vi "ProfiledPIDController_Calculate_Meas_StateGoal.vi"(9 "GoalState":T1 {"Velocity" format="%16_6e"; "Position" format="%16_6e"}, 10 "PV-Measurement":dbl, 11 "in PROFILED_PID_CONTROLLER":T2={"Controller"={"Kp"=0.0, "Ki"=0.0, "Kd"=0.0, "Period"=0.0, "Max_Integral"=1.0, "Min_Integral"=-1.0, "Max_Input"=0.0, "Min_Input"=0.0, "Continuous"=FALSE, "PositionError"=0.0, "VelocityError"=0.0, "PrevError"=0.0, "TotalError"=0.0, "PositionTolerance"=0.05, "VelocityTolerance"=9.99e+35, "SetPoint"=0.0, "Kf"=0.0, "Prev_Deriv"=0.0, "Prev_Deriv 2"=0.0, "DerivativeFilter"=FALSE, "Min_Output"=-9.99e+35, "Max_Output"=9.9e+35, "Prev_F_P"=0.0, "Prev_F_P_2"=0.0, "AntiWindupActive"=FALSE}, "Goal"={"Position"=0.0, "Velocity"=0.0}, "Setpoint"={"Position"=0.0, "Velocity"=0.0}, "Constraint"={"MaxVelocity"=0.0, "MaxAcceleration"=0.0}} {"Constraint"."MaxAcceleration" format="%16_6e"; "Constraint"."MaxVelocity" format="%16_6e"; "Setpoint"."Velocity" format="%16_6e"; "Setpoint"."Position" format="%16_6e"; "Goal"."Velocity" format="%16_6e"; "Goal"."Position" format="%16_6e"; "Controller"."Prev_F_P_2" format="%16_6e"; "Controller"."Prev_F_P" format="%16_6e"; "Controller"."Max_Output" format="%16_6e"; "Controller"."Min_Output" format="%16_6e"; "Controller"."Prev_Deriv 2" format="%16_6e"; "Controller"."Prev_Deriv" format="%16_6e"; "Controller"."Kf" format="%16_6e"; "Controller"."SetPoint" format="%16_6e"; "Controller"."VelocityTolerance" format="%16_6e"; "Controller"."PositionTolerance" format="%16_6e"; "Controller"."TotalError" format="%16_6e"; "Controller"."PrevError" format="%16_6e"; "Controller"."VelocityError" format="%16_6e"; "Controller"."PositionError" format="%16_6e"; "Controller"."Min_Input" format="%16_6e"; "Controller"."Max_Input" format="%16_6e"; "Controller"."Min_Integral" format="%16_6e"; "Controller"."Max_Integral" format="%16_6e"; "Controller"."Period" format="%16_6e"; "Controller"."Kd" format="%16_6e"; "Controller"."Ki" format="%16_6e"; "Controller"."Kp" format="%16_6e"}) -> (1 "CO-ControlOutput":dbl, 3 "out PROFILED_PID_CONTROLLER":T2={"Controller"={"Kp"=0.0, "Ki"=0.0, "Kd"=0.0, "Period"=0.0, "Max_Integral"=1.0, "Min_Integral"=-1.0, "Max_Input"=0.0, "Min_Input"=0.0, "Continuous"=FALSE, "PositionError"=0.0, "VelocityError"=0.0, "PrevError"=0.0, "TotalError"=0.0, "PositionTolerance"=0.05, "VelocityTolerance"=9.99e+35, "SetPoint"=0.0, "Kf"=0.0, "Prev_Deriv"=0.0, "Prev_Deriv 2"=0.0, "DerivativeFilter"=FALSE, "Min_Output"=-9.99e+35, "Max_Output"=9.9e+35, "Prev_F_P"=0.0, "Prev_F_P_2"=0.0, "AntiWindupActive"=FALSE}, "Goal"={"Position"=0.0, "Velocity"=0.0}, "Setpoint"={"Position"=0.0, "Velocity"=0.0}, "Constraint"={"MaxVelocity"=0.0, "MaxAcceleration"=0.0}} {"Constraint"."MaxAcceleration" format="%16_6e"; "Constraint"."MaxVelocity" format="%16_6e"; "Setpoint"."Velocity" format="%16_6e"; "Setpoint"."Position" format="%16_6e"; "Goal"."Velocity" format="%16_6e"; "Goal"."Position" format="%16_6e"; "Controller"."Prev_F_P_2" format="%16_6e"; "Controller"."Prev_F_P" format="%16_6e"; "Controller"."Max_Output" format="%16_6e"; "Controller"."Min_Output" format="%16_6e"; "Controller"."Prev_Deriv 2" format="%16_6e"; "Controller"."Prev_Deriv" format="%16_6e"; "Controller"."Kf" format="%16_6e"; "Controller"."SetPoint" format="%16_6e"; "Controller"."VelocityTolerance" format="%16_6e"; "Controller"."PositionTolerance" format="%16_6e"; "Controller"."TotalError" format="%16_6e"; "Controller"."PrevError" format="%16_6e"; "Controller"."VelocityError" format="%16_6e"; "Controller"."PositionError" format="%16_6e"; "Controller"."Min_Input" format="%16_6e"; "Controller"."Max_Input" format="%16_6e"; "Controller"."Min_Integral" format="%16_6e"; "Controller"."Max_Integral" format="%16_6e"; "Controller"."Period" format="%16_6e"; "Controller"."Kd" format="%16_6e"; "Controller"."Ki" format="%16_6e"; "Controller"."Kp" format="%16_6e"})   [LabVIEW 2019, in "Trajectory_Library.lvlib"]
doc: "Returns the next output of the PID controller.\n\nInputs:\n - Profiled_PID_Controller -- Profiled_PID_Controller data cluster\n - measurement -- The current measurement of the process variable.\n - goal -- The new goal of the controller.\n\nOutputs:\n - Profiled_PID_Controller -- Updated Profiled_PID_Controller data cluster\n - CO-ControlOutput -- Calculated PID output"
uses:
  Trajectory_Library.lvlib
  PID_CONTROLLER.ctl
  TRAPEZOID_PROFILE_STATE.ctl
  TRAPEZOID_PROFILE_CONSTRAINT.ctl
  PROFILED_PID_CONTROLLER.ctl
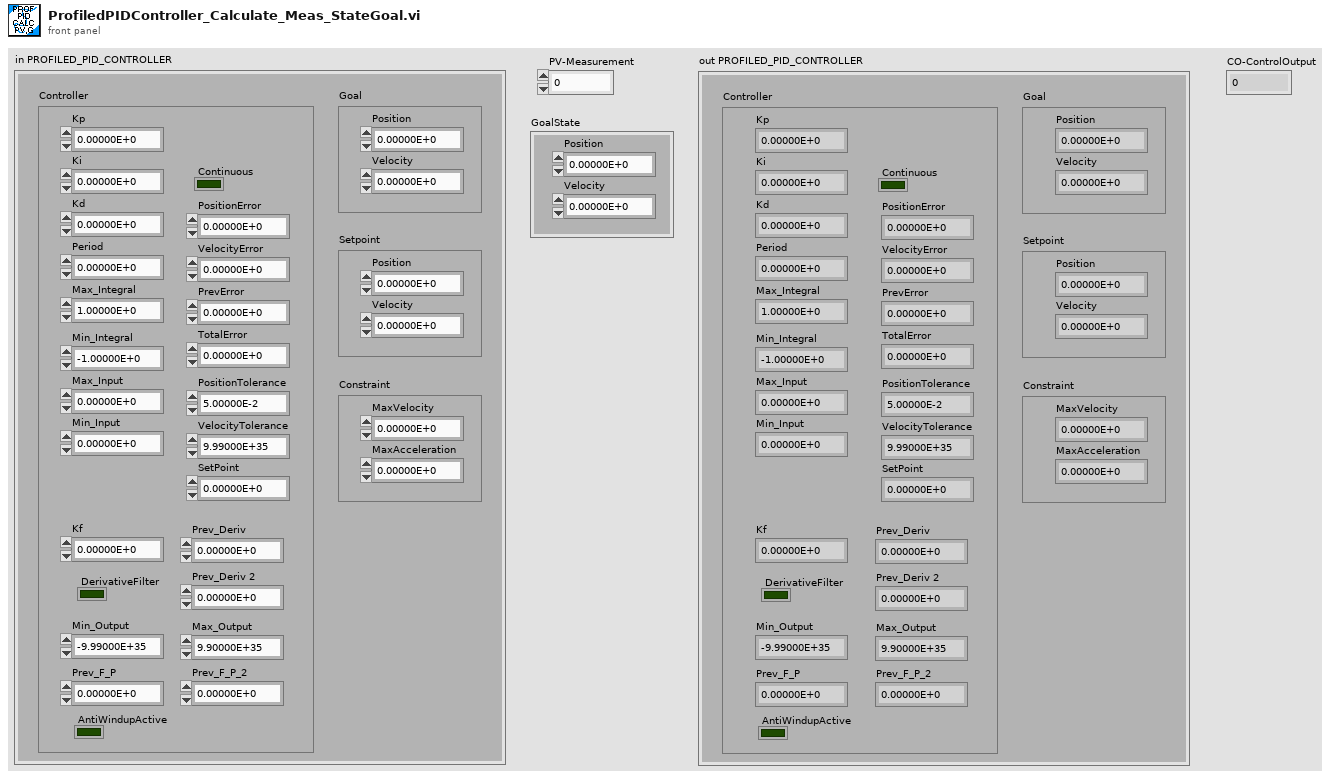
[diagram p1: front panel]
types:
  T1 = typedef "Trajectory_Library.lvlib/TRAPEZOID_PROFILE_STATE.ctl" = cluster{"Position":dbl, "Velocity":dbl}
  T2 = typedef "Trajectory_Library.lvlib/PROFILED_PID_CONTROLLER.ctl" = cluster{"Controller":T3, "Goal":T1, "Setpoint":T1, "Constraint":T4}
  T3 = typedef "Trajectory_Library.lvlib/PID_CONTROLLER.ctl" = cluster{"Kp":dbl, "Ki":dbl, "Kd":dbl, "Period":dbl, "Max_Integral":dbl, "Min_Integral":dbl, "Max_Input":dbl, "Min_Input":dbl, "Continuous":bool, "PositionError":dbl, "VelocityError":dbl, "PrevError":dbl, "TotalError":dbl, "PositionTolerance":dbl, "VelocityTolerance":dbl, "SetPoint":dbl, "Kf":dbl, "Prev_Deriv":dbl, "Prev_Deriv 2":dbl, "DerivativeFilter":bool, "Min_Output":dbl, "Max_Output":dbl, "Prev_F_P":dbl, "Prev_F_P_2":dbl, "AntiWindupActive":bool}
  T4 = typedef "Trajectory_Library.lvlib/TRAPEZOID_PROFILE_CONSTRAINT.ctl" = cluster{"MaxVelocity":dbl, "MaxAcceleration":dbl}
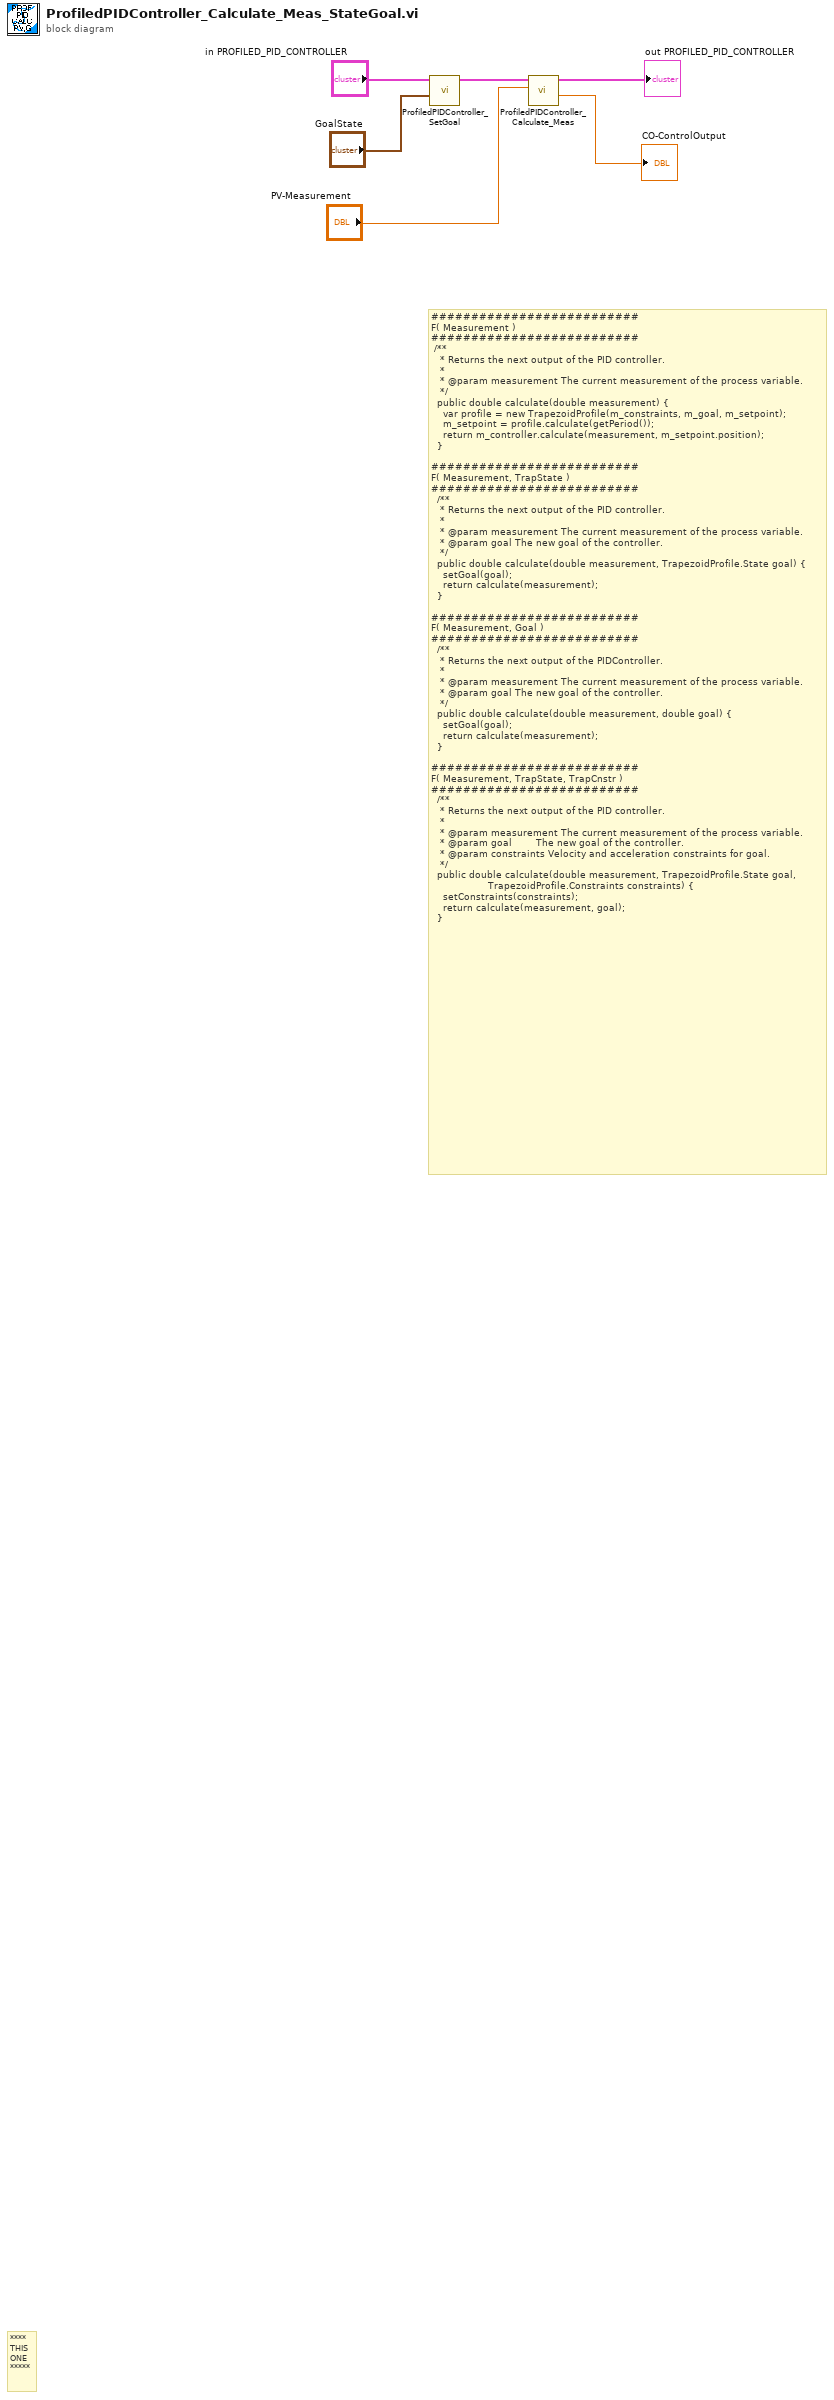
[diagram p0: block diagram]
diagram:
  # "##########################\nF( Measurement ) \n##########################\n /**\n   * Returns the next output of the PID controller.\n   *\n   * @param measurement The current measurement of the process variable.\n   */\n  public double calculate(double measurement) {\n    var profile = new TrapezoidProfile(m_constraints, m_goal, m_setpoint);\n    m_setpoint = profile.calculate(getPeriod());\n    return m_controller.calculate(measurement, m_setpoint.position);\n  }\n\n##########################\nF( Measurement, TrapState ) \n##########################\n  /**\n   * Returns the next output of the PID controller.\n   *\n   * @param measurement The current measurement of the process variable.\n   * @param goal The new goal of the controller.\n   */\n  public double calculate(double measurement, TrapezoidProfile.State goal) {\n    setGoal(goal);\n    return calculate(measurement);\n  }\n\n##########################\nF( Measurement, Goal ) \n##########################\n  /**\n   * Returns the next output of the PIDController.\n   *\n   * @param measurement The current measurement of the process variable.\n   * @param goal The new goal of the controller.\n   */\n  public double calculate(double measurement, double goal) {\n    setGoal(goal);\n    return calculate(measurement);\n  }\n\n##########################\nF( Measurement, TrapState, TrapCnstr ) \n##########################\n  /**\n   * Returns the next output of the PID controller.\n   *\n   * @param measurement The current measurement of the process variable.\n   * @param goal        The new goal of the controller.\n   * @param constraints Velocity and acceleration constraints for goal.\n   */\n  public double calculate(double measurement, TrapezoidProfile.State goal,\n                   TrapezoidProfile.Constraints constraints) {\n    setConstraints(constraints);\n    return calculate(measurement, goal);\n  }"
  # "****\nTHIS\nONE\n*****"
  n1 = call "ProfiledPIDController_SetGoal.vi"("Goal"="GoalState", "in PROFILED_PID_CONTROLLER"="in PROFILED_PID_CONTROLLER") -> ("out PROFILED_PID_CONTROLLER"=w5:T2)  [unwired: 9 in]
  n2 = call "ProfiledPIDController_Calculate_Meas.vi"("PV-Measurement"="PV-Measurement", "in PROFILED_PID_CONTROLLER"=w5) -> ("CO-ControlOutput"=→"CO-ControlOutput":dbl, "out PROFILED_PID_CONTROLLER"=→"out PROFILED_PID_CONTROLLER":T2)  [unwired: 8 in]
